vi "Test data.vi"(11 "Error in":errorcluster) -> (15 "Error out":errorcluster)   [LabVIEW 2020, in "Database Tests.lvlib"]
doc: "This VI is used for validating database search"
uses:
  Database Tests.lvlib
  typedefs/account details array.ctl
  typedefs/card number search result.ctl
  typedefs/card_numbers.ctl
  typedefs/valid upto search result array.ctl
  typedefs/card holder name search result array.ctl
  <vilib>/addons/_JKI Toolkits/Caraya/classes/Test Suite/Define Test Suite (JUnit Report).vi
  <vilib>/SLL Drona/APIs/Stimulus/ControlValue/SetValueAuto.vi
  <vilib>/SLL Drona/APIs/Assert/AssertControlValue/Equal.vi
  <vilib>/SLL Drona/APIs/Stimulus/VI/CloseVI.vi
  <vilib>/Utility/error.llb/Error Cluster From Error Code.vi
  <vilib>/ErrorRing/Error Ring.xnode
  <vilib>/addons/_JKI Toolkits/Caraya/classes/Test Suite/Test Suite.lvclass
  <vilib>/addons/_JKI Toolkits/Caraya/classes/Test/Test.lvclass
  <vilib>/SLL Drona/Drona.lvlib
  <vilib>/SLL Drona/APIs/Stimulus/ControlValue/ControlValue.lvlib
  <vilib>/SLL Drona/APIs/Assert/AssertControlValue/AssertControlValue.lvlib
  <vilib>/Wiresmith Technology/G CLI/CLI Class/CLI.lvclass
  <vilib>/SLL Drona/APIs/Stimulus/VI/VI.lvlib
panel:
  # "TEST DATA"
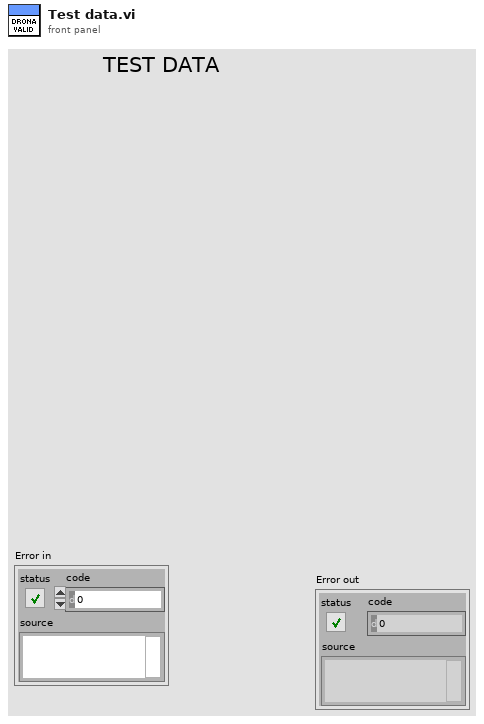
[diagram p1: front panel]
types:
  T1 = typedef "Database Tests.lvlib/account details array.ctl" = cluster{"Card Number":i64, "Card Holder Name":string, "Valid upto":i32}[]
  T2 = typedef "Database Tests.lvlib/card number search result.ctl" = cluster{"Card Number":dbl, "Card Holder Name":string, "Vaild upto":dbl}
  T3 = typedef "Database Tests.lvlib/card_numbers.ctl" = enum16{"Card Holder Name", "Card Number", "Valid upto"}
  T4 = typedef "Database Tests.lvlib/valid upto search result array.ctl" = cluster{"Card Number":dbl, "Card Holder Name":string, "Valid upto":dbl}[]
  T5 = typedef "Database Tests.lvlib/card holder name search result array.ctl" = T2[]
  T6 = cluster{"Account Details":T1, "Card Holder Name":string, "Card Number":i64, "Card Number Search result":T2, "Search option":T3, "Vaild upto":i32, "Valid Upto Serach Result":T4, "Search option 2":T3, "Search option 3":T3, "Card Number Search Result Array":T5}[]
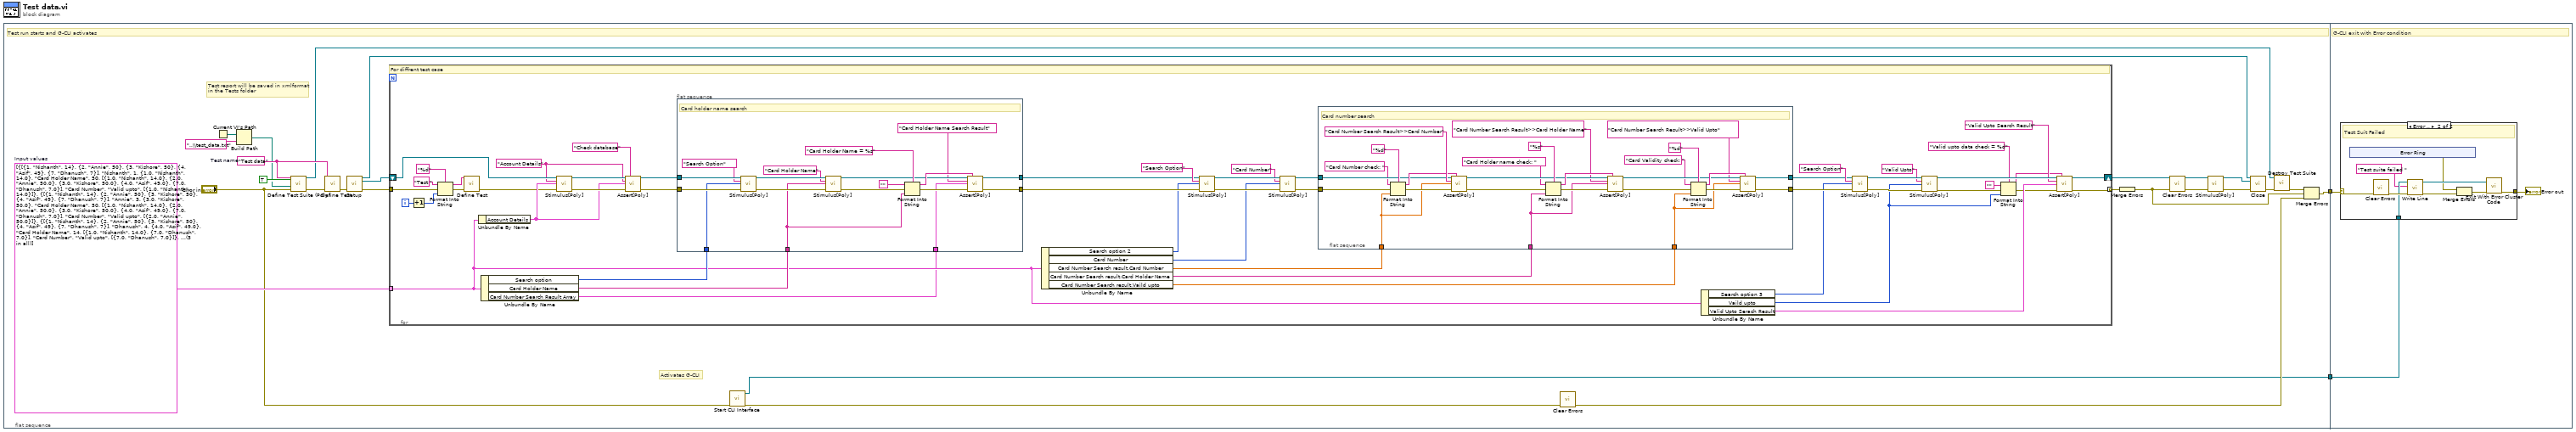
[diagram p0: block diagram]
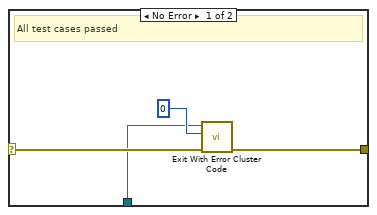
[diagram p2: hidden frame]
diagram:
  n1 = flat-sequence {
    tunnel: [w17] -> w2
    tunnel: [w8] -> w1
    tunnel: w2 -> [w125]
    tunnel: w1 -> [w123]
    frame #0 {
      w23 = T6 [{"Account Details"=[{"Card Number"=1, "Card Holder Name"="Nishanth", "Valid upto"=14}, {"Card Number"=2, "Card Holder Name"="Annie", "Valid upto"=50}, {"Card Number"=3, "Card Holder Name"="Kishore", "Valid upto"=50}, {"Card Number"=4, "Card Holder Name"="Asif", "Valid upto"=49}, {"Card Number"=7, "Card Holder Name"="Dhanush", "Valid upto"=7}], "Card Holder Name"="Nishanth", "Card Number"=1, "Card Number Search result"={"Card Number"=1.0, "Card Holder Name"="Nishanth", "Vaild upto"=14.0}, "Search option"=enum."Card Holder Name", "Vaild upto"=50, "Valid Upto Serach Result"=[{"Card Number"=1.0, "Card Holder Name"="Nishanth", "Valid upto"=14.0}, {"Card Number"=2.0, "Card Holder Name"="Annie", "Valid upto"=50.0}, {"Card Number"=3.0, "Card Holder Name"="Kishore", "Valid upto"=50.0}, {"Card Number"=4.0, "Card Holder Name"="Asif", "Valid upto"=49.0}, {"Card Number"=7.0, "Card Holder Name"="Dhanush", "Valid upto"=7.0}], "Search option 2"=enum."Card Number", "Search option 3"=enum."Valid upto", "Card Number Search Result Array"=[{"Card Number"=1.0, "Card Holder Name"="Nishanth", "Vaild upto"=14.0}]}, {"Account Details"=[{"Card Number"=1, "Card Holder Name"="Nishanth", "Valid upto"=14}, {"Card Number"=2, "Card Holder Name"="Annie", "Valid upto"=50}, {"Card Number"=3, "Card Holder Name"="Kishore", "Valid upto"=50}, {"Card Number"=4, "Card Holder Name"="Asif", "Valid upto"=49}, {"Card Number"=7, "Card Holder Name"="Dhanush", "Valid upto"=7}], "Card Holder Name"="Annie", "Card Number"=3, "Card Number Search result"={"Card Number"=3.0, "Card Holder Name"="Kishore", "Vaild upto"=50.0}, "Search option"=enum."Card Holder Name", "Vaild upto"=50, "Valid Upto Serach Result"=[{"Card Number"=1.0, "Card Holder Name"="Nishanth", "Valid upto"=14.0}, {"Card Number"=2.0, "Card Holder Name"="Annie", "Valid upto"=50.0}, {"Card Number"=3.0, "Card Holder Name"="Kishore", "Valid upto"=50.0}, {"Card Number"=4.0, "Card Holder Name"="Asif", "Valid upto"=49.0}, {"Card Number"=7.0, "Card Holder Name"="Dhanush", "Valid upto"=7.0}], "Search option 2"=enum."Card Number", "Search option 3"=enum."Valid upto", "Card Number Search Result Array"=[{"Card Number"=2.0, "Card Holder Name"="Annie", "Vaild upto"=50.0}]}, {"Account Details"=[{"Card Number"=1, "Card Holder Name"="Nishanth", "Valid upto"=14}, {"Card Number"=2, "Card Holder Name"="Annie", "Valid upto"=50}, {"Card Number"=3, "Card Holder Name"="Kishore", "Valid upto"=50}, {"Card Number"=4, "Card Holder Name"="Asif", "Valid upto"=49}, {"Card Number"=7, "Card Holder Name"="Dhanush", "Valid upto"=7}], "Card Holder Name"="Dhanush", "Card Number"=4, "Card Number Search result"={"Card Number"=4.0, "Card Holder Name"="Asif", "Vaild upto"=49.0}, "Search option"=enum."Card Holder Name", "Vaild upto"=14, "Valid Upto Serach Result"=[{"Card Number"=1.0, "Card Holder Name"="Nishanth", "Valid upto"=14.0}, {"Card Number"=7.0, "Card Holder Name"="Dhanush", "Valid upto"=7.0}], "Search option 2"=enum."Card Number", "Search option 3"=enum."Valid upto", "Card Number Search Result Array"=[{"Card Number"=7.0, "Card Holder Name"="Dhanush", "Vaild upto"=7.0}]}]  # Input values
      w14 = "Test data"  # Test name
      # "Test report will be saved in xmlformat\nin the Tests folder"
      # "Activates G-CLI"
      # "Test run starts and G-CLI activates"
      n2 = Current VI's Path() -> (path=w12:path)
      n3 = Build Path(base path=w12, name or relative path="..\\test_data.txt") -> (appended path=w10:path)
      n4 = call-poly <vilib>:"Define Test Suite (Poly).vi"("error in (no error)"="Error in", "Report Path"=w10, "Interactive"=TRUE, "Label (VI Title)"=w14) -> ("error out"=w16:errorcluster, "Test Suite"=w5:refnum<class "Test Suite.lvclass">)  [unwired: 5 in, 1 out]
      n5 = call <vilib>:"Define Test.vi"("error in (no error)"=w16, "Label (VI Title)"=w14) -> ("error out"=w27:errorcluster)  [unwired: 8 in, 1 out]
      n6 = call <vilib>:"Setup.vi"("error in"=w27) -> ("Application Ref"=w25:refnum<vi>, "VI Reference Out"=w24:refnum<vi>, "error out"=w26:errorcluster)  [unwired: 12 in]
      n7 = for {
        tunnel: w23 -> [w57] mode=indexing
        shift-right: [w51] -> w22
        shift-left: w24 -> [w49]
        tunnel: w26 -> [w36]
        tunnel: [w54] -> w19 mode=indexing
        i -> [w32]
        w39 = "Account Details" ("Control Path")
        # "For diffrent test case"
        n8 = Increment(x=w32) -> (x+1=w29:i32)
        n9 = Format Into String(format string="%d", initial string="Test ", error in=w36, w29) -> (resulting string=w31:string, error out=w35:errorcluster)
        n10 = call <vilib>:"Define Test.vi"("error in (no error)"=w35, "Label (VI Title)"=w31) -> ("error out"=w30:errorcluster)  [unwired: 8 in, 1 out]
        n11 = Unbundle By Name(w57) -> ("Account Details"=w38:T1)
        n12 = Unbundle By Name(w57) -> ("Search option"=w78:T3, "Card Holder Name"=w77:string, "Card Number Search Result Array"=w28:T5)
        n13 = call-poly <vilib>:"Stimulus[Poly].vi"("VI Reference In"=w49, "Control Path"=w39, "Value (Signaling)"=w38, "error in"=w30) -> ("VI Reference Out"=w40:refnum<vi>, "error out"=w43:errorcluster)  [unwired: 10 in]
        n14 = call-poly <vilib>:"Assert[Poly].vi"("VI Reference In"=w40, "Test Label"="Check database", "Control Path"=w39, "Control Value"=w38, "Error In"=w43) -> ("VI Reference Out"=w41:refnum<vi>, "Error Out"=w42:errorcluster)  [unwired: 9 in]
        n15 = flat-sequence {
          tunnel: w42 -> [w122]
          tunnel: w41 -> [w121]
          tunnel: w78 -> [w120]
          tunnel: w77 -> [w106]
          tunnel: [w110] -> w73
          tunnel: [w111] -> w71
          tunnel: w28 -> [w105]
          frame #0 {
            # "Card holder name search"
            n16 = call-poly <vilib>:"Stimulus[Poly].vi"("VI Reference In"=w121, "Control Path"="Search Option", "Value (Signaling)"=w120, "error in"=w122) -> ("VI Reference Out"=w117:refnum<vi>, "error out"=w118:errorcluster)  [unwired: 10 in]
            n17 = call-poly <vilib>:"Stimulus[Poly].vi"("VI Reference In"=w117, "Control Path"="Card Holder Name", "Value (Signaling)"=w106, "error in"=w118) -> ("VI Reference Out"=w108:refnum<vi>, "error out"=w112:errorcluster)  [unwired: 10 in]
            n18 = Format Into String(format string="Card Holder Name = %s", initial string="", error in=w112, w106) -> (resulting string=w113:string, error out=w109:errorcluster)
            n19 = call-poly <vilib>:"Assert[Poly].vi"("VI Reference In"=w108, "Test Label"=w113, "Control Path"="Card Holder Name Search Result", "Control Value"=w105, "Error In"=w109) -> ("VI Reference Out"=w111:refnum<vi>, "Error Out"=w110:errorcluster)  [unwired: 9 in]
          }
        }
        n20 = Unbundle By Name(w57) -> ("Search option 2"=w70:T3, "Card Number"=w67:i64, "Card Number Search result.Card Number"=w66:dbl, "Card Number Search result.Card Holder Name"=w65:string, "Card Number Search result.Vaild upto"=w64:dbl)
        n21 = call-poly <vilib>:"Stimulus[Poly].vi"("VI Reference In"=w71, "Control Path"="Search Option", "Value (Signaling)"=w70, "error in"=w73) -> ("VI Reference Out"=w74:refnum<vi>, "error out"=w75:errorcluster)  [unwired: 10 in]
        n22 = call-poly <vilib>:"Stimulus[Poly].vi"("VI Reference In"=w74, "Control Path"="Card Number", "Value (Signaling)"=w67, "error in"=w75) -> ("VI Reference Out"=w68:refnum<vi>, "error out"=w69:errorcluster)  [unwired: 10 in]
        n23 = flat-sequence {
          tunnel: [w90] -> w59
          tunnel: w69 -> [w84]
          tunnel: w68 -> [w83]
          tunnel: w66 -> [w81]
          tunnel: w65 -> [w92]
          tunnel: w64 -> [w88]
          tunnel: [w86] -> w58
          frame #0 {
            # "Card number search"
            n24 = Format Into String(format string="%d", initial string="Card Number check: ", error in=w84, w81) -> (resulting string=w101:string, error out=w104:errorcluster)
            n25 = call-poly <vilib>:"Assert[Poly].vi"("VI Reference In"=w83, "Test Label"=w101, "Control Path"="Card Number Search Result>>Card Number", "Control Value"=w81, "Error In"=w104) -> ("VI Reference Out"=w94:refnum<vi>, "Error Out"=w100:errorcluster)  [unwired: 9 in]
            n26 = Format Into String(format string="%s", initial string="Card Holder name check: ", error in=w100, w92) -> (resulting string=w95:string, error out=w97:errorcluster)
            n27 = call-poly <vilib>:"Assert[Poly].vi"("VI Reference In"=w94, "Test Label"=w95, "Control Path"="Card Number Search Result>>Card Holder Name", "Control Value"=w92, "Error In"=w97) -> ("VI Reference Out"=w87:refnum<vi>, "Error Out"=w96:errorcluster)  [unwired: 9 in]
            n28 = Format Into String(format string="%d", initial string="Card Validity check: ", error in=w96, w88) -> (resulting string=w89:string, error out=w91:errorcluster)
            n29 = call-poly <vilib>:"Assert[Poly].vi"("VI Reference In"=w87, "Test Label"=w89, "Control Path"="Card Number Search Result>>Valid Upto", "Control Value"=w88, "Error In"=w91) -> ("VI Reference Out"=w86:refnum<vi>, "Error Out"=w90:errorcluster)  [unwired: 9 in]
          }
        }
        n30 = Unbundle By Name(w57) -> ("Search option 3"=w56:T3, "Vaild upto"=w52:i32, "Valid Upto Serach Result"=w53:T4)
        n31 = call-poly <vilib>:"Stimulus[Poly].vi"("VI Reference In"=w58, "Control Path"="Search Option", "Value (Signaling)"=w56, "error in"=w59) -> ("VI Reference Out"=w61:refnum<vi>, "error out"=w62:errorcluster)  [unwired: 10 in]
        n32 = call-poly <vilib>:"Stimulus[Poly].vi"("VI Reference In"=w61, "Control Path"="Valid Upto", "Value (Signaling)"=w52, "error in"=w62) -> ("VI Reference Out"=w50:refnum<vi>, "error out"=w55:errorcluster)  [unwired: 10 in]
        n33 = Format Into String(format string="Valid upto data check = %d", initial string="", error in=w55, w52) -> (resulting string=w47:string, error out=w46:errorcluster)
        n34 = call-poly <vilib>:"Assert[Poly].vi"("VI Reference In"=w50, "Test Label"=w47, "Control Path"="Valid Upto Search Result", "Control Value"=w53, "Error In"=w46) -> ("VI Reference Out"=w51:refnum<vi>, "Error Out"=w54:errorcluster)  [unwired: 9 in]
      }
      n35 = call <vilib>:"Start CLI Interface.vi"("error in (no error)"="Error in") -> ("error out"=w9:errorcluster, "CLI out"=w8:refnum<class "CLI.lvclass">)  [unwired: 7 in, 2 out]
      n36 = call <vilib>:"Clear Errors.vi"("error in (no error)"=w9) -> ("error out"=w18:errorcluster)  [unwired: 5 in, 1 out]
      n37 = Merge Errors(w19) -> (w3:errorcluster)
      n38 = call <vilib>:"Clear Errors.vi"("error in (no error)"=w3) -> ("error out"=w4:errorcluster)  [unwired: 5 in, 1 out]
      n39 = call-poly <vilib>:"Stimulus[Poly].vi"("VI Reference In"=w22, "error in"=w4) -> ("VI Reference Out"=w20:refnum<vi>, "error out"=w21:errorcluster)  [unwired: 12 in]
      n40 = call <vilib>:"Close.vi"("Application Ref"=w25, "VI Reference"=w20, "error in"=w21) -> ("error out"=w7:errorcluster)  [unwired: 12 in]
      n41 = call-dynamic "Destroy Test Suite.vi"("error in (no error)"=w7, "Test Suite in"=w5) -> ("error out"=w6:errorcluster)  [unwired: 8 in, 1 out]
      n42 = Merge Errors(w6, w3, w18) -> (w17:errorcluster)
    }
    frame #1 {
      # "G-CLI exit with Error condition"
      n43 = case shown="Error .." w125 {
        selector: w125 -> [w129 w137]
        tunnel: [w128 w138] -> w124
        tunnel: w123 -> [w126 w131]
        frame No Error {
          # "All test cases passed"
          n44 = call <vilib>:"Exit With Error Cluster Code.vi"("error in (no error)"=w129, "No Error Code (0)"=0, "CLI in"=w126) -> ("error out"=w128:errorcluster)  [unwired: 8 in]
        }
        frame Error {
          # "Test Suit Failed"
          n45 = xnode "Error Ring"() -> ("error out"=w133:errorcluster)
          n46 = call <vilib>:"Clear Errors.vi"("error in (no error)"=w137) -> ("error out"=w136:errorcluster)  [unwired: 5 in, 1 out]
          n47 = call <vilib>:"Write Line.vi"("error in (no error)"=w136, "Text to Write"="Test suite failed ", "CLI in"=w131) -> ("error out"=w132:errorcluster, "CLI out"=w135:refnum<class "CLI.lvclass">)  [unwired: 7 in]
          n48 = Merge Errors(w133, w132) -> (w134:errorcluster)
          n49 = call <vilib>:"Exit With Error Cluster Code.vi"("error in (no error)"=w134, "CLI in"=w135) -> ("error out"=w138:errorcluster)  [unwired: 9 in]
        }
      }
      "Error out" <- w124
    }
  }
